vi "Cleanup.vi"(0 "Operation Interface in":refnum<class "Program Interface.lvclass">) -> ()   [LabVIEW 2016, in "Program Interface.lvclass"]
uses:
  Program Interface.lvclass
  Program Interface.lvclass/Program Interface.ctl
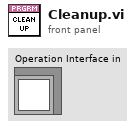
[diagram p1: front panel]
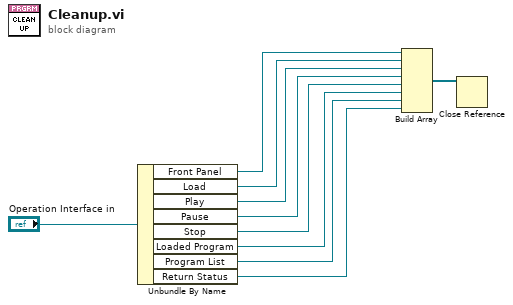
[diagram p0: block diagram]
diagram:
  n1 = Unbundle By Name("Operation Interface in") -> ("Front Panel"=w9:refnum<vi>, "Load"=w8:refnum<vi>, "Play"=w7:refnum<vi>, "Pause"=w6:refnum<vi>, "Stop"=w5:refnum<vi>, "Loaded Program"=w4:refnum<vi>, "Program List"=w3:refnum<vi>, "Return Status"=w2:refnum<vi>)
  n2 = Build Array(w9, w8, w7, w6, w5, w4, w3, w2) -> (w1:refnum<vi>[])
  n3 = Close Reference(reference=w1) -> ()  [unwired: 1 in, 1 out]
